vi "Keith 7001 Send Message.vi"(2 "timeout ms":u32=4294967295 format="%.0x", 3 "address string":string, 4 "write buffer":string, 7 "source":string, 8 "write mode (set END:0)":i32(ring) items=["send EOI with last character of string", "append CR to string and send EOI with CR", "append LF to string and send EOI with LF", "append CR LF to string and send EOI with LF", "append CR to string but do not send EOI", "append LF to string but do not send EOI", "append CR LF to string but do not send EOI", "do not send EOI"], 9 "error in":T1) -> (0 "address out":string, 1 "byte count":i32, 5 "status":bool[](array[boolean]), 6 "error out":T1)   [LabVIEW 2019]
doc: "Sends a string to a message based VXI instrument. In order to communicate with an instrument, you must first open the instrument by running the Open VXI Instrument or running the initialize VI (initialize VIs call the Open VXI Instrument in their block diagram). Use the instrument ID generated by the Open VXI Instrument to address the specific instrument, then set the write mode and enter the string to send. If a write error occurs, error code 1230 is returned. If you fail to open the instrument, error code 1232 is returned."
panel:
  in  "[empty array]":bool[](array[boolean])
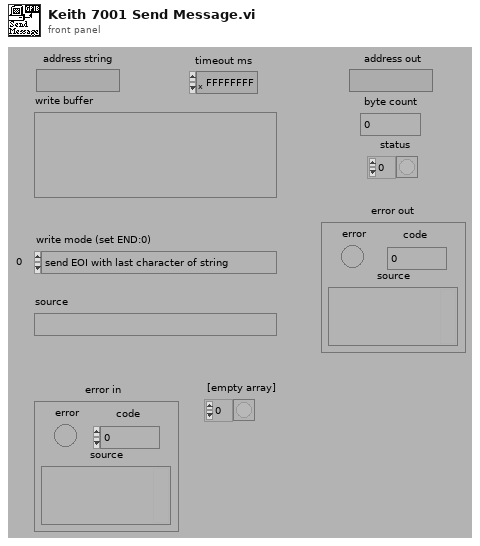
[diagram p1: front panel]
types:
  T1 = cluster{"error":bool, "code":i32, "source":string}
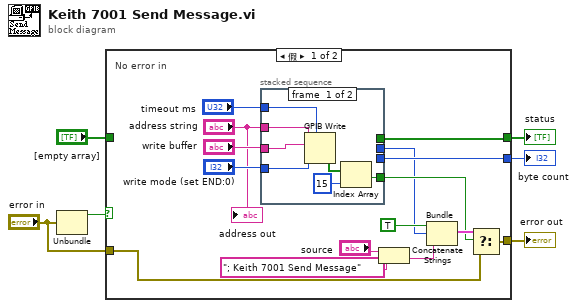
[diagram p0: block diagram]
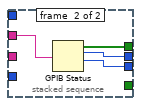
[diagram p2: hidden frame]
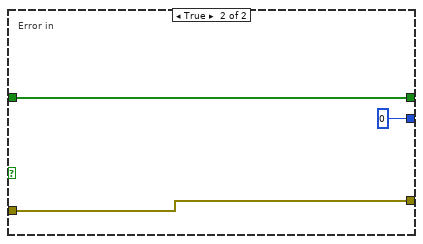
[diagram p3: hidden frame]
diagram:
  n1 = Unbundle("error in") -> ("error"=w4:bool)  [unwired: 2 out]
  n2 = case shown="假" w4 {
    tunnel: "[empty array]" -> [_ w33]
    tunnel: [w14 w33] -> w5
    tunnel: [w20 w34] -> w1
    tunnel: "error in" -> [w11 w34]
    tunnel: [w15 0] -> w6
    frame False {
      # "No error in"
      n3 = stacked-sequence {
        tunnel: [_ w31] -> w14
        tunnel: [_ w32] -> w15
        tunnel: [w25 _] -> w16
        tunnel: "write mode (set END:0)" -> [w22 _]
        tunnel: "write buffer" -> [w26 _]
        tunnel: [_ w30] -> w13
        tunnel: "address string" -> [w24 w29]
        tunnel: "timeout ms" -> [w23 _]
        frame #0 {
          n4 = GPIB Write(0:w24, 1:w26, 2:w22, 4:w23) -> (5:w27:bool[])  [unwired: 1 in, 1 out]
          n5 = Index Array(array=w27, index=15) -> (element=w25:bool)
        }
        frame #1 {
          n6 = GPIB Status(0:w29) -> (2:w31:bool[], 3:w30:i16, 4:w32:i32)  [unwired: 1 in, 1 out]
        }
      }
      n7 = Concatenate Strings("source", "; Keith 7001 Send Message") -> (w12:string)
      n8 = Bundle(TRUE, "GPIB error"=w13, w12) -> (w21:cluster{bool, "GPIB error":i16, string})  [unwired: 1 in]
      n9 = Select(t=w21, s=w16, f=w11) -> (s? t:f=w20:T1)
      "address out" <- "address string"
    }
    frame True {
      # "Error in"
    }
  }
  "status" <- w5
  "byte count" <- w6
  "error out" <- w1
